vi "Find Templates.vi"() -> (1 "Template Path":path, 2 "List Folders":string[](array[string]))   [LabVIEW 2025, in "_Template.lvlib" / "_Template.lvclass"]
uses:
  _Template.lvclass
  _Template.lvclass/_Template.ctl
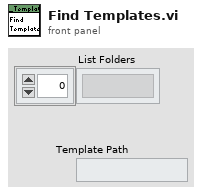
[diagram p1: front panel]
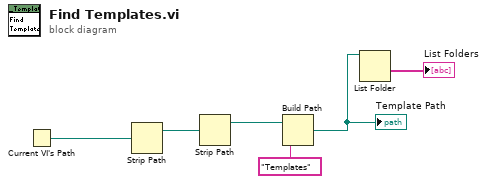
[diagram p0: block diagram]
diagram:
  n1 = Current VI's Path() -> (path=w4:path)
  n2 = Strip Path(path=w4) -> (stripped path=w3:path)  [unwired: 1 out]
  n3 = Strip Path(path=w3) -> (stripped path=w2:path)  [unwired: 1 out]
  n4 = Build Path(base path=w2, name or relative path="Templates" ("regular expression")) -> (appended path=w5:path)
  "Template Path" <- w5
  n5 = List Folder(path=w5) -> (folder names=→"List Folders":string[])  [unwired: 3 in, 3 out]
